vi "Exercise 3-6.vi"() -> ()   [LabVIEW 2014]
panel:
  out "output":dbl
  in  "input":dbl
  in  "Enum":T1(ring)
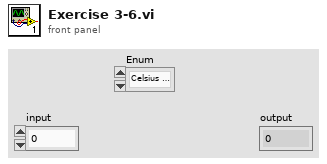
[diagram p1: front panel]
types:
  T1 = enum16{"Celsius to Fahrenheit", "Fahrenheit to Celsius", "Celsius to Kelvin", "Fahrenheit to Kelvin"}
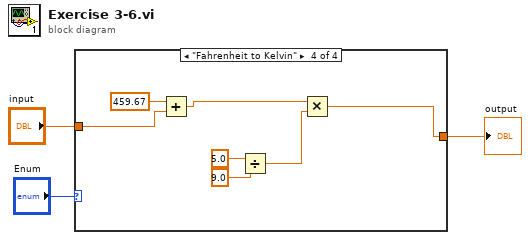
[diagram p0: block diagram]
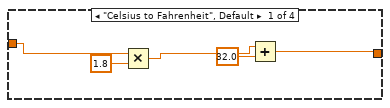
[diagram p2: hidden frame]
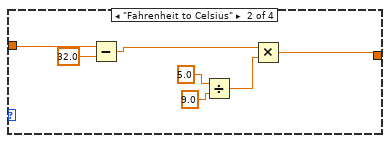
[diagram p3: hidden frame]
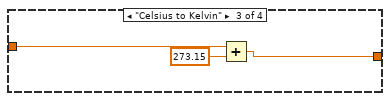
[diagram p4: hidden frame]
diagram:
  n1 = case shown="\"Fahrenheit to Kelvin\"" "Enum" {
    tunnel: "input" -> [w8 w15 w18 w19]
    tunnel: [w4 w13 w17 w21] -> w1
    frame "Celsius to Fahrenheit", Default {
      n2 = Multiply(x=w8, y=1.8) -> (x*y=w6:dbl)
      n3 = Add(x=w6, y=32.0) -> (x+y=w4:dbl)
    }
    frame "Fahrenheit to Celsius" {
      n4 = Subtract(x=w15, y=32.0) -> (x-y=w14:dbl)
      n5 = Divide(x=5.0, y=9.0) -> (x/y=w11:dbl)
      n6 = Multiply(x=w14, y=w11) -> (x*y=w13:dbl)
    }
    frame "Celsius to Kelvin" {
      n7 = Add(x=w18, y=273.15) -> (x+y=w17:dbl)
    }
    frame "Fahrenheit to Kelvin" {
      n8 = Add(x=459.67, y=w19) -> (x+y=w22:dbl)
      n9 = Divide(x=5.0, y=9.0) -> (x/y=w23:dbl)
      n10 = Multiply(x=w22, y=w23) -> (x*y=w21:dbl)
    }
  }
  "output" <- w1
